vi "Run Service.vi"(10 "reentrant":bool=TRUE, 11 "server settings":T1) -> (0 "error out":errorcluster)   [LabVIEW 2021, in "MeasurementServerTests.lvlib" / "Measurement Service Tests.lvlib" / "Continuous Counting Measurement.lvclass"]
uses:
  Continuous Counting Measurement.lvclass
  Runtime/Measurements/Helpers/TypeDefs/Measurement Server User Settings.ctl
  Runtime/Measurements/Helpers/TypeDefs/Stop Server User Event.ctl
  Runtime/Measurements/Helpers/TypeDefs/Measurement Service Version.ctl
  C:/Dev/github/ni/measurementlink-labview/Source/Runtime/Measurements/Measurement Plugin Service/Measurement Plugin Service.lvclass
  _Measurement Logic.vi
  Runtime/Measurements/NI Measurement Plug-In SDK.lvlib
panel:
  # "Run this VI to start the measurement service.  A window will appear that provides basic information about the running service.\n\nUse the stop button on the window that appears to stop the measurement service."
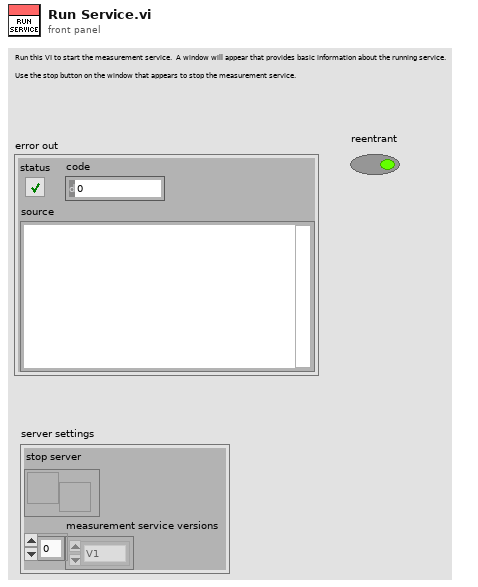
[diagram p1: front panel]
types:
  T1 = typedef "NI Measurement Plug-In SDK.lvlib/Measurement Server User Settings.ctl" = cluster{"stop server":T2, "measurement service versions":T3[]}
  T2 = typedef "NI Measurement Plug-In SDK.lvlib/Stop Server User Event.ctl" = refnum<user-event>
  T3 = typedef "NI Measurement Plug-In SDK.lvlib/Measurement Service Version.ctl" = enum16{"V1", "V2"}
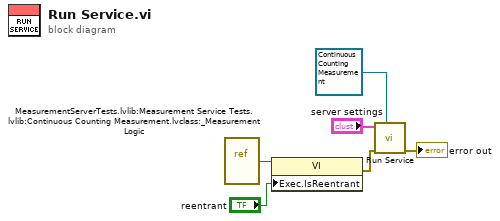
[diagram p0: block diagram]
diagram:
  n1 = vi-ref "MeasurementServerTests.lvlib:Measurement Service Tests.lvlib:Continuous Counting Measurement.lvclass:_Measurement Logic.vi"() -> (w4:refnum<vi>)
  n2 = property class="VI"(reference=w4, "Exec.IsReentrant"="reentrant") -> (error out=w2:errorcluster)  [unwired: 1 in, 1 out]
  n3 = call "Run Service.vi"("measurement"=refnum<class "Continuous Counting Measurement.lvclass"> refnum ("MeasurementServerTests.lvlib:Measurement Plugin Service Tests.lvlib:Continuous Counting Measurement.lvclass"), "error in"=w2, "measurementlink server user settings"="server settings") -> ("error out"=→"error out":errorcluster)  [unwired: 8 in]
